vi "TOOLweb SET LABFILE BaseName.vi"(4 "error in (no error)":errorcluster, 5 "IP-Adresse (localhost)":string="127.0.0.1", 7 "BaseName":string) -> (0 "error out":errorcluster caption="Fehler (Ausgang)", 1 "Feedback":i32, 3 "Neuer Name":string)   [LabVIEW 2020, in "FT-IR.lvlib" / "TOOLweb Interface.lvlib"]
doc: "Ändert den ersten Teil des Dateinamens für die \"labfiles\" mit einem SET-Request (EVID 82) und gibt die Antwort des Messgerätes in \"Neuer Name\" wieder. \nDer Integer-Ausgang \"Feedback\" gibt Auskunft über die erfolgreiche Ausführung des Set-Requests, wobei nur der Wert 0 (=success) für alle EVIDs gleich ist. Fehlermeldungen in Form einer Feedback-Zahl ungleich Null variieren und müssen mit dem Handbuch des Gas-Analysators interpretiert werden.\n\nFalls der TOOLWeb-Server nicht auf demselben Rechner arbeitet, kann mit \"IP-Adresse\" eine beliebiger Host adressiert werden. Ein unverbundener Eingang spricht den lokalen Host an."
uses:
  TOOLweb Interface.lvlib
  Stoerungen/Stoerungen Messgeraet/Aktionen Kommunikation Stoerung.ctl
  Stoerungen/Stoerungen.lvlib
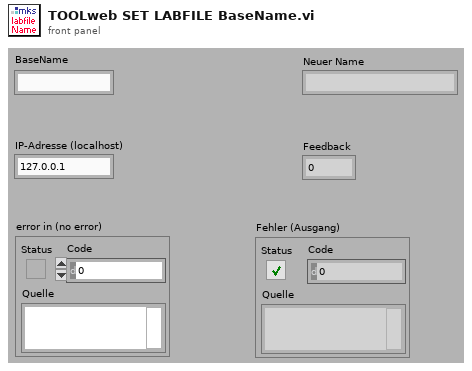
[diagram p1: front panel]
types:
  T1 = typedef "Stoerungen.lvlib/Aktionen Kommunikation Stoerung.ctl" = enum16{"lesen", "init", "FT-IR Komm", "FT-IR Betriebsart", "FT-IR Hintergrund", "cRIO Komm", "PNS Komm", "Dichtheitstest", "Life Bit", "FTIR Komm AK", "PMA Komm", "FID Komm", "PMA Cal", "FID Ch4 Cal", "FID THC Cal", "Cal Timeout", "VFS 1 Komm", "VFS 2 Komm", "VFS 3 Komm", "VFS 4 Komm", "TRE 08 Komm", "CG-Test vorzeitig", "CG-Test Span 1", "CG-Test Span 2", "CG-Test Span 3", "CG-Test Messgas", "CG-Test löschen", "Test", "Amium AK", "AK Recept konfig", "AK Name konfig", "AK EKFG konfig"}
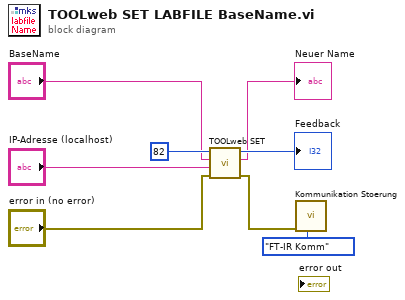
[diagram p0: block diagram]
diagram:
  n1 = call "TOOLweb SET.vi"("error in (no error)"="error in (no error)", "IP-Adresse (localhost)"="IP-Adresse (localhost)", "Wert-String"="BaseName", "EVID-Nummer"=82) -> ("error out"=w1:errorcluster, "Neuer Wert"=→"Neuer Name":string, "Feedback"=→"Feedback":i32)  [unwired: 1 out]
  n2 = call "Kommunikation Stoerung.vi"("Aktionen"=Aktionen_Kommunikation_Stoerung."FT-IR Komm", "error in"=w1) -> ()  [unwired: 9 in, 1 out]
